vi "Shutdown.vi"(11 "Sound Demo in":refnum<class "Sound Demo.lvclass">) -> (0 "error out":errorcluster, 3 "Sound Demo out":refnum<class "Sound Demo.lvclass">)   [LabVIEW 2017, in "Sound Demo.lvclass"]
doc: "Shutdown the sound player."
uses:
  Sound Demo.lvclass
  Sound Demo.lvclass/Sound Demo.ctl
  Sound Player/Sound Player.lvclass
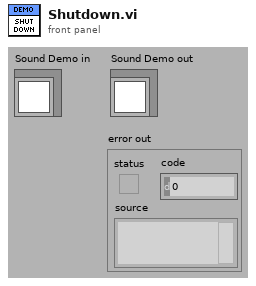
[diagram p1: front panel]
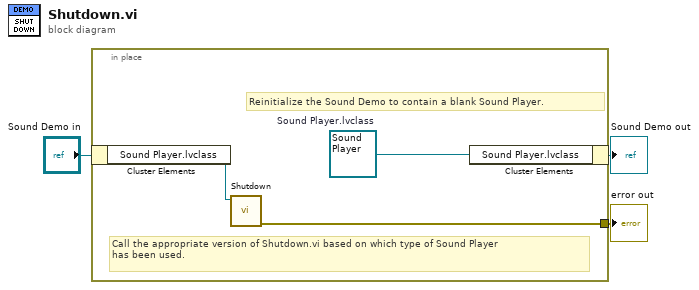
[diagram p0: block diagram]
diagram:
  n1 = in-place {
    in-place-border: [w4] -> w1
    w5 = refnum<class "Sound Player.lvclass"> refnum  # Sound Player.lvclass
    # "Call the appropriate version of Shutdown.vi based on which type of Sound Player \nhas been used."
    # "Reinitialize the Sound Demo to contain a blank Sound Player."
    n2 = in-place-cluster #1("Sound Demo in") -> ("Sound Player.lvclass"=w6:refnum<class "Sound Player.lvclass">)
    n3 = call-dynamic "Shutdown.vi"("Sound Player in"=w6) -> ("error out"=w4:errorcluster)  [unwired: 9 in, 1 out]
    n4 = in-place-cluster #1("Sound Player.lvclass"=w5) -> (→"Sound Demo out":refnum<class "Sound Demo.lvclass">)
  }
  "error out" <- w1
